vi "Replace VI Contents.vi"(8 "error in (no error)":errorcluster, 9 "Target VI":path, 10 "Template VI":path, 11 "Application":refnum<vi>) -> (0 "error out":errorcluster, 1 "Target vi refnum":refnum<vi>, 3 "Application":refnum<vi>)   [LabVIEW 2019, in "BlueUtilityScripts.lvlib"]
uses:
  BlueUtilityScripts.lvlib
  <vilib>/Utility/miscctls.llb/LVPositionTypeDef.ctl
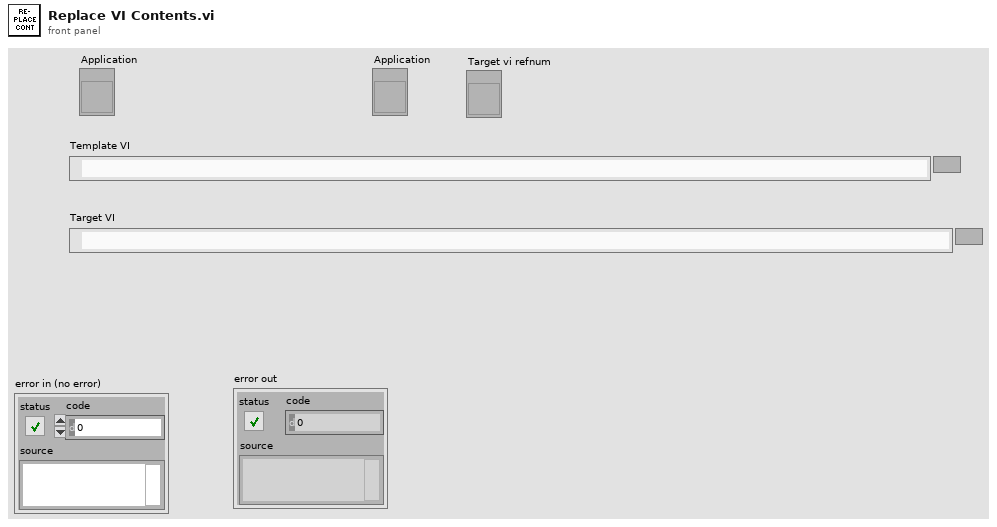
[diagram p1: front panel]
types:
  T1 = typedef "LVPositionTypeDef.ctl" = cluster{"Left":i32, "Top":i32}
  T2 = enum16{"Invalid Wire Rule", "Required", "Recommended", "Optional", "Dynamic Dispatch"}[]
  T3 = enum16{"Invalid Wire Rule", "Required", "Recommended", "Optional", "Dynamic Dispatch"}
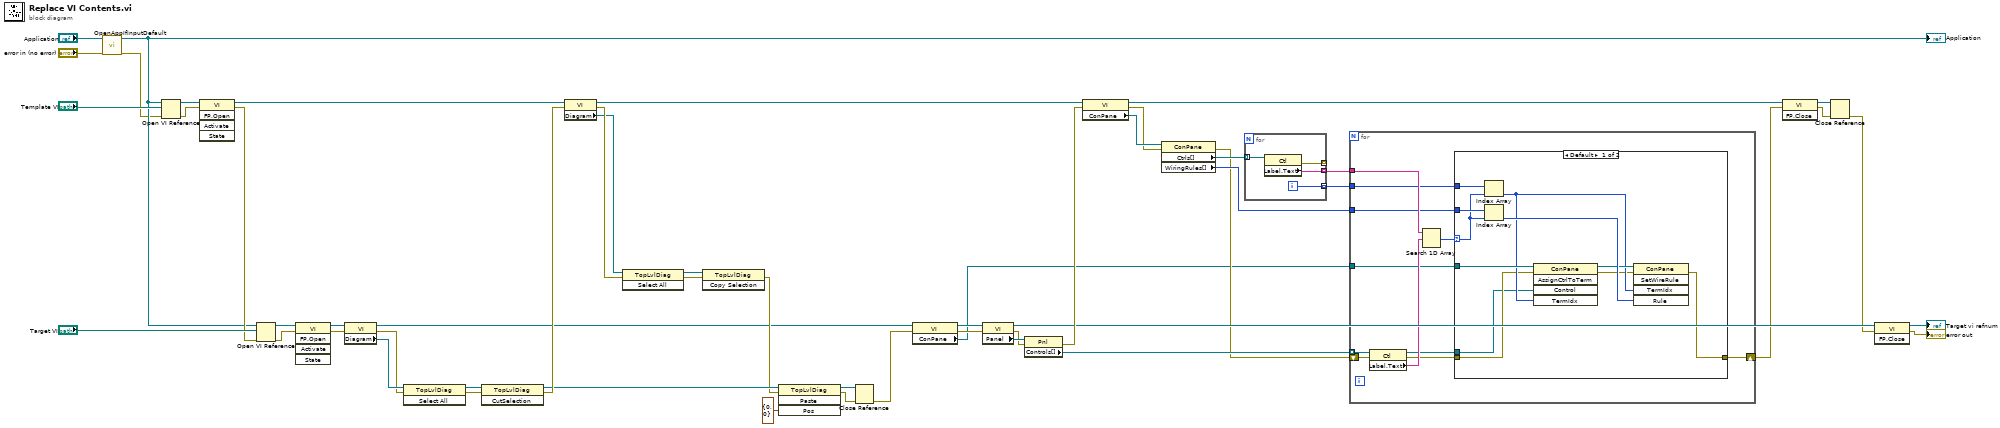
[diagram p0: block diagram]
diagram:
  n1 = call "OpenAppIfInputDefault.vi"("error in (no error)"="error in (no error)", "Application"="Application") -> ("error out"=w4:errorcluster, "valid application reference"=w6:refnum<vi>)  [unwired: 7 in, 1 out]
  "Application" <- w6
  n2 = Open VI Reference(application reference (local)=w6, vi path="Template VI", error in (no error)=w4) -> (vi reference=w35:refnum<vi>, error out=w34:errorcluster)  [unwired: 3 in]
  n3 = invoke class="VI" method="FP.Open"(reference=w35, error in=w34) -> (reference out=w33:refnum<vi>, error out=w16:errorcluster)  [unwired: 3 in, 3 out]
  n4 = Open VI Reference(application reference (local)=w6, vi path="Target VI", error in (no error)=w16) -> (vi reference=w51:refnum<vi>, error out=w47:errorcluster)  [unwired: 3 in]
  n5 = invoke class="VI" method="FP.Open"(reference=w51, error in=w47) -> (reference out=w50:refnum<vi>, error out=w46:errorcluster)  [unwired: 3 in, 3 out]
  n6 = property class="VI"(reference=w50, error in=w46) -> (reference out=w25:refnum<vi>, error out=w45:errorcluster, "Diagram"=w49:refnum<vi>)
  n7 = invoke class="TopLvlDiag" method="Select All"(reference=w49, error in=w45) -> (reference out=w48:refnum<vi>, error out=w44:errorcluster)  [unwired: 1 in, 1 out]
  n8 = invoke class="TopLvlDiag" method="CutSelection"(reference=w48, error in=w44) -> (reference out=w40:refnum<vi>, error out=w41:errorcluster)  [unwired: 1 in, 1 out]
  n9 = property class="VI"(reference=w33, error in=w41) -> (reference out=w32:refnum<vi>, error out=w43:errorcluster, "Diagram"=w42:refnum<vi>)
  n10 = invoke class="TopLvlDiag" method="Select All"(reference=w42, error in=w43) -> (reference out=w39:refnum<vi>, error out=w36:errorcluster)  [unwired: 1 in, 1 out]
  n11 = invoke class="TopLvlDiag" method="Copy Selection"(reference=w39, error in=w36) -> (error out=w38:errorcluster)  [unwired: 1 in, 2 out]
  n12 = invoke class="TopLvlDiag" method="Paste"(reference=w40, error in=w38, "Pos"=T1 {"Left"=0, "Top"=0} ("Position")) -> (reference out=w22:refnum<vi>, error out=w21:errorcluster)  [unwired: 1 in, 2 out]
  n13 = Close Reference(reference=w22, error in (no error)=w21) -> (error out=w20:errorcluster)
  n14 = property class="VI"(reference=w25, error in=w20) -> (reference out=w23:refnum<vi>, error out=w19:errorcluster, "ConPane"=w1:refnum<vi>)
  n15 = property class="VI"(reference=w23, error in=w19) -> (reference out=w11:refnum<vi>, error out=w18:errorcluster, "Panel"=w29:refnum<vi>)
  n16 = property class="Pnl"(reference=w29, error in=w18) -> (error out=w17:errorcluster, "Controls[]"=w28:refnum<vi>[])  [unwired: 1 out]
  n17 = property class="VI"(reference=w32, error in=w17) -> (reference out=w14:refnum<vi>, error out=w15:errorcluster, "ConPane"=w31:refnum<vi>)
  n18 = property class="ConPane"(reference=w31, error in=w15) -> (error out=w3:errorcluster, "Ctrls[]"=w30:refnum<vi>[], "WiringRules[]"=w24:T2)  [unwired: 1 out]
  n19 = for {
    tunnel: w30 -> [w57] mode=indexing
    tunnel: [w56] -> w27 mode=indexing
    tunnel: [w55] -> w26 mode=indexing
    tunnel: [w54] -> _ mode=indexing
    i -> [w55]
    n20 = property class="Ctl"(reference=w57) -> (error out=w54:errorcluster, "Label.Text"=w56:string)  [unwired: 1 in, 1 out]
  }
  n21 = for {
    tunnel: w28 -> [w68] mode=indexing
    tunnel: w27 -> [w67]
    tunnel: w26 -> [w65]
    tunnel: w24 -> [w64]
    shift-right: [w59] -> w2
    shift-left: w3 -> [w61]
    tunnel: w1 -> [w58]
    n22 = property class="Ctl"(reference=w68, error in=w61) -> (reference out=w62:refnum<vi>, error out=w60:errorcluster, "Label.Text"=w63:string)
    n23 = Search 1D Array(1D array=w67, element=w63) -> (index of element=w66:i32)  [unwired: 1 in]
    n24 = case shown="Default" w66 {
      selector: w66 -> [w77 _]
      tunnel: w58 -> [w75 _]
      tunnel: w65 -> [w79 _]
      tunnel: w64 -> [w78 _]
      tunnel: w62 -> [w69 _]
      tunnel: w60 -> [w72 w80]
      tunnel: [w70 w80] -> w59
      frame Default {
        n25 = Index Array(array=w79, index=w77) -> (element=w73:i32)
        n26 = Index Array(array=w78, index=w77) -> (element=w76:T3)
        n27 = invoke class="ConPane" method="AssignCtrlToTerm"(reference=w75, error in=w72, "Control"=w69, "TermIdx"=w73) -> (reference out=w74:refnum<vi>, error out=w71:errorcluster)  [unwired: 1 in, 3 out]
        n28 = invoke class="ConPane" method="SetWireRule"(reference=w74, error in=w71, "TermIdx"=w73, "Rule"=w76) -> (error out=w70:errorcluster)  [unwired: 1 in, 4 out]
      }
      frame -1 {
      }
    }
  }
  n29 = invoke class="VI" method="FP.Close"(reference=w14, error in=w2) -> (reference out=w13:refnum<vi>, error out=w12:errorcluster)  [unwired: 1 in, 1 out]
  n30 = Close Reference(reference=w13, error in (no error)=w12) -> (error out=w9:errorcluster)
  n31 = invoke class="VI" method="FP.Close"(reference=w11, error in=w9) -> (reference out=→"Target vi refnum":refnum<vi>, error out=→"error out":errorcluster)  [unwired: 1 in, 1 out]
